vi "Set Build Exclusions.vi"(9 "Build specification name":string="Configuration - Release", 10 "target name":string="My Computer", 11 "Source project":path=path "C:/SE/Custom Devices/Scan Engine and EtherCAT/Custom Device Source/Scan Engine.lvproj") -> (0 "error out":errorcluster)   [LabVIEW 2010]
uses:
  <vilib>/AppBuilder/AB_API/SDIST/NI_AB_API_SDIST.lvclass
  <vilib>/AppBuilder/AB_API/common/AB_API Primary Exclusions.ctl
  <vilib>/AppBuilder/AB_API/DSDIST/NI_AB_API_DSDIST.lvclass
  <vilib>/AppBuilder/AB_API/common/AB_API Build Object Type.ctl
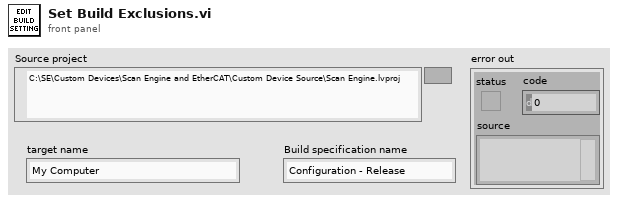
[diagram p1: front panel]
types:
  T1 = typedef "AB_API Build Object Type.ctl" = enum16{"Source Distribution", "DLL", "EXE", "Installer", "Zip File", "RESTful WS", "RTEXE", "Packed Library", "C Generation "}
  T2 = typedef "AB_API Primary Exclusions.ctl" = cluster{"Disconnect type definitions":bool, "Remove unused polymorphic VI instances":bool, "Remove unused members of project libraries":bool, "Modify project library file after removing unused members":bool}
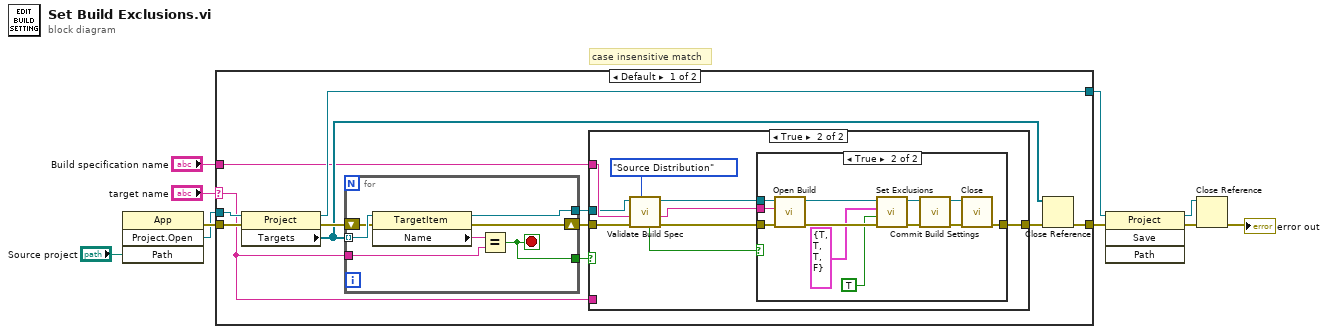
[diagram p0: block diagram]
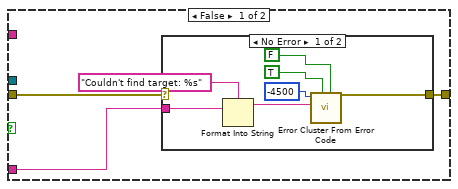
[diagram p2: hidden frame]
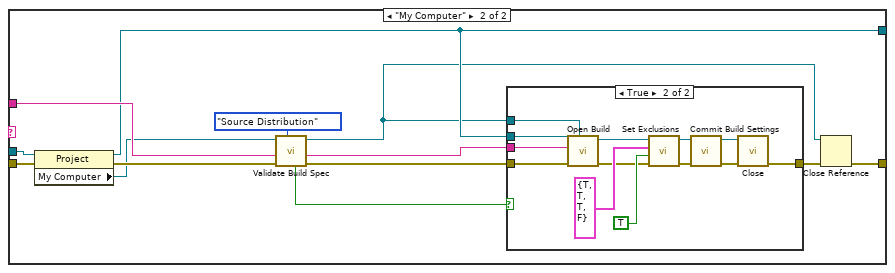
[diagram p5: hidden frame]
diagram:
  # "case insensitive match"
  n1 = invoke class="App" method="Project.Open"("Path"="Source project") -> (error out=w4:errorcluster, "Project:Open"=w3:refnum<vi>)  [unwired: 3 in, 2 out]
  n2 = case shown="Default" "target name" {
    selector: "target name" -> [w11 _]
    tunnel: [w17 w65] -> w10
    tunnel: w4 -> [w19 w74]
    tunnel: "Build specification name" -> [w14 w72]
    tunnel: w3 -> [w20 w70]
    tunnel: [w18 w69] -> w2
    frame Default {
      n3 = property class="Project"(reference=w20, error in=w19) -> (reference out=w18:refnum<vi>, error out=w21:errorcluster, "Targets"=w16:refnum<vi>[])
      n4 = for {
        tunnel: w16 -> [w62] mode=indexing
        shift-right: [w60] -> w15
        shift-left: w21 -> [w61]
        tunnel: w11 -> [w58]
        tunnel: [w57] -> w13
        tunnel: [w56] -> w12
        stop <- w56 stop-if-true
        n5 = property class="TargetItem"(reference=w62, error in=w61) -> (reference out=w57:refnum<vi>, error out=w60:errorcluster, "Name"=w59:string)
        n6 = Equal?(x=w59, y=w58) -> (x = y?=w56:bool)
      }
      n7 = case shown="True" w12 {
        tunnel: [w25 w42] -> w22
        tunnel: w15 -> [w24 w41]
        tunnel: w14 -> [_ w39]
        tunnel: w13 -> [_ w38]
        tunnel: w11 -> [w23 _]
        frame False {
          n8 = case shown="No Error" w24 {
            selector: w24 -> [_ w33]
            tunnel: [w32 w33] -> w25
            tunnel: w23 -> [w31 _]
            frame No Error {
              n9 = Format Into String(format string="Couldn't find target: %s", w31) -> (resulting string=w28:string)  [unwired: 2 in, 1 out]
              n10 = call <vilib>:"Error Cluster From Error Code.vi"("is warning? (False)"=FALSE, "show call chain? (False)"=TRUE, "error message (\"\")"=w28, "error code (0)"=-4500) -> ("error out"=w32:errorcluster)  [unwired: 5 in]
            }
            frame Error {
            }
          }
        }
        frame True {
          n11 = call "Validate Build Spec.vi"("Build object type"=AB_API_Build_Object_Type."Source Distribution", "error in (no error)"=w41, "Build spec name"=w39, "TargetItem in"=w38) -> ("error out"=w40:errorcluster, "Build spec name dup"=w36:string, "TargetItem out"=w37:refnum<vi>, "Valid"=w34:bool)  [unwired: 4 in]
          n12 = case shown="True" w34 {
            tunnel: [w43 w50] -> w42
            tunnel: w40 -> [w43 w48]
            tunnel: w37 -> [_ w47]
            tunnel: w36 -> [_ w46]
            frame False {
            }
            frame True {
              n13 = call <vilib>:"Open Build.vi"("error in (no error)"=w48, "Build specification name"=w46, "TargetItem Refnum"=w47) -> ("error out"=w55:errorcluster, "DSDIST out"=w54:refnum<class "NI_AB_API_DSDIST.lvclass">)  [unwired: 7 in]
              n14 = call-dynamic "Set Exclusions.vi"("error in (no error)"=w55, "Disconnect inline subVIs"=TRUE, "Exclusions"=T2 {"Disconnect type definitions"=TRUE, "Remove unused polymorphic VI instances"=TRUE, "Remove unused members of project libraries"=TRUE, "Modify project library file after removing unused members"=FALSE}, "SDIST in"=w54) -> ("error out"=w49:errorcluster, "SDIST out"=w53:refnum<class "NI_AB_API_DSDIST.lvclass">)  [unwired: 6 in]
              n15 = call-dynamic "Commit Build Settings.vi"("error in (no error)"=w49, "DSDIST in"=w53) -> ("error out"=w51:errorcluster, "DSDIST out"=w52:refnum<class "NI_AB_API_DSDIST.lvclass">)  [unwired: 8 in]
              n16 = call-dynamic "Close.vi"("error in (no error)"=w51, "SDIST in"=w52) -> ("error out"=w50:errorcluster)  [unwired: 9 in]
            }
          }
        }
      }
      n17 = Close Reference(reference=w16, error in (no error)=w22) -> (error out=w17:errorcluster)
    }
    frame "My Computer" {
      n18 = property class="Project"(reference=w70, error in=w74) -> (reference out=w69:refnum<vi>, error out=w71:errorcluster, "My Computer"=w68:refnum<vi>)
      n19 = call "Validate Build Spec.vi"("Build object type"=AB_API_Build_Object_Type."Source Distribution", "error in (no error)"=w71, "Build spec name"=w72, "TargetItem in"=w68) -> ("error out"=w73:errorcluster, "Build spec name dup"=w67:string, "TargetItem out"=w64:refnum<vi>, "Valid"=w63:bool)  [unwired: 4 in]
      n20 = case shown="True" w63 {
        tunnel: [w76 w85] -> w75
        tunnel: w73 -> [w76 w83]
        tunnel: w69 -> [_ w82]
        tunnel: w67 -> [_ w81]
        tunnel: w64 -> [_ w77]
        frame False {
        }
        frame True {
          n21 = call <vilib>:"Open Build.vi"("TargetItem Refnum"=w77, "error in (no error)"=w83, "Build specification name"=w81, "Project Refnum"=w82) -> ("error out"=w78:errorcluster, "SDIST out"=w84:refnum<class "NI_AB_API_SDIST.lvclass">)  [unwired: 6 in]
          n22 = call-dynamic "Set Exclusions.vi"("error in (no error)"=w78, "Disconnect inline subVIs"=TRUE, "Exclusions"=T2 {"Disconnect type definitions"=TRUE, "Remove unused polymorphic VI instances"=TRUE, "Remove unused members of project libraries"=TRUE, "Modify project library file after removing unused members"=FALSE}, "SDIST in"=w84) -> ("error out"=w88:errorcluster, "SDIST out"=w89:refnum<class "NI_AB_API_SDIST.lvclass">)  [unwired: 6 in]
          n23 = call-dynamic "Commit Build Settings.vi"("error in (no error)"=w88, "SDIST in"=w89) -> ("error out"=w86:errorcluster, "SDIST out"=w87:refnum<class "NI_AB_API_SDIST.lvclass">)  [unwired: 8 in]
          n24 = call-dynamic "Close.vi"("error in (no error)"=w86, "SDIST in"=w87) -> ("error out"=w85:errorcluster)  [unwired: 9 in]
        }
      }
      n25 = Close Reference(reference=w64, error in (no error)=w75) -> (error out=w65:errorcluster)
    }
  }
  n26 = invoke class="Project" method="Save"(reference=w2, error in=w10) -> (reference out=w8:refnum<vi>, error out=w9:errorcluster)  [unwired: 2 in, 2 out]
  n27 = Close Reference(reference=w8, error in (no error)=w9) -> (error out=→"error out":errorcluster)
